vi "add glyph core.vi"(6 "image data":T1, 8 "error in":errorcluster, 9 "name":string, 10 "base glyphs":T1[](array[typedef]), 11 "map in":variant) -> (0 "error out":errorcluster, 2 "base glyphs out":T1[](array[typedef]), 3 "map out":variant)   [LabVIEW 2013, in "glyph manager.lvlib"]
uses:
  glyph manager.lvlib
  <vilib>/picture/picture.llb/imagedata.ctl
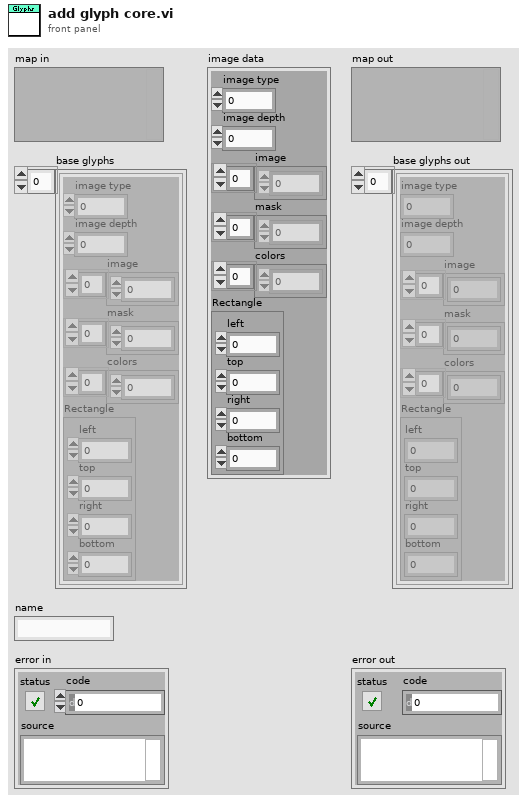
[diagram p1: front panel]
types:
  T1 = typedef "imagedata.ctl" = cluster{"image type":i32, "image depth":i32, "image":u8[], "mask":u8[], "colors":u32[], "Rectangle":cluster{"left":i16, "top":i16, "right":i16, "bottom":i16}}
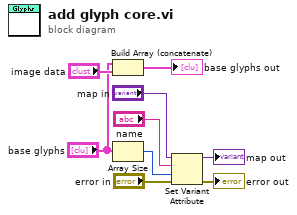
[diagram p0: block diagram]
diagram:
  n1 = Build Array (concatenate)("base glyphs", "image data") -> (→"base glyphs out":T1[])
  n2 = Array Size(array="base glyphs") -> (size(s)=w4:i32)
  n3 = Set Variant Attribute(Variant="map in", name="name", value=w4, error in="error in") -> (Variant out=→"map out":variant, error out=→"error out":errorcluster)  [unwired: 1 out]
